vi "New User (popup).vi"(0 "file path (use dialog)":path, 11 "error in (no error)":errorcluster) -> (15 "error out":errorcluster)   [LabVIEW 2012]
uses:
  SubVIs/typedef/User Accounts.ctl
panel:
  out "Info Password not secure":bool
  out "Stop App?":bool
  in  "Cancel":bool
  in  "User\nName":string
  in  "Password":string
  in  "Rewrite\nPassword":string
  in  "Admin":bool
  in  "Create":bool
  # "Log In attempt"
  # "of"
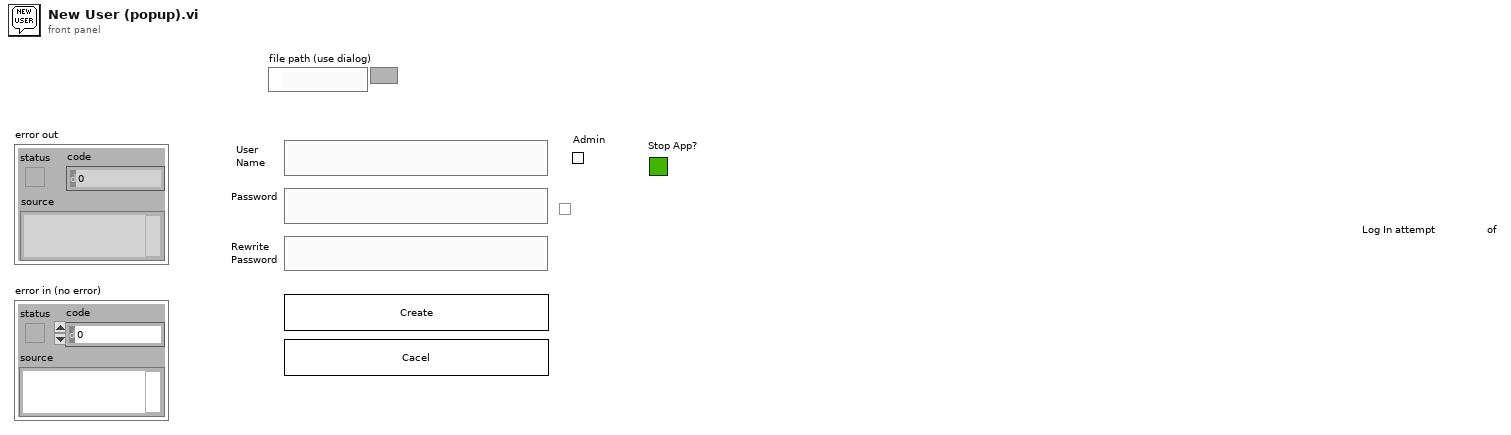
[diagram p1: front panel]
types:
  T1 = typedef "User Accounts.ctl" = enum16{"None", "User", "Admin"}
  T2 = cluster{"Usuario":string, "Password":string, "Account type":T1}
  T3 = typedef "User_Data_Cluster.ctl" = cluster{"Usuario":string, "Password":string, "Account type":T1, "Time Stamp":timestamp}
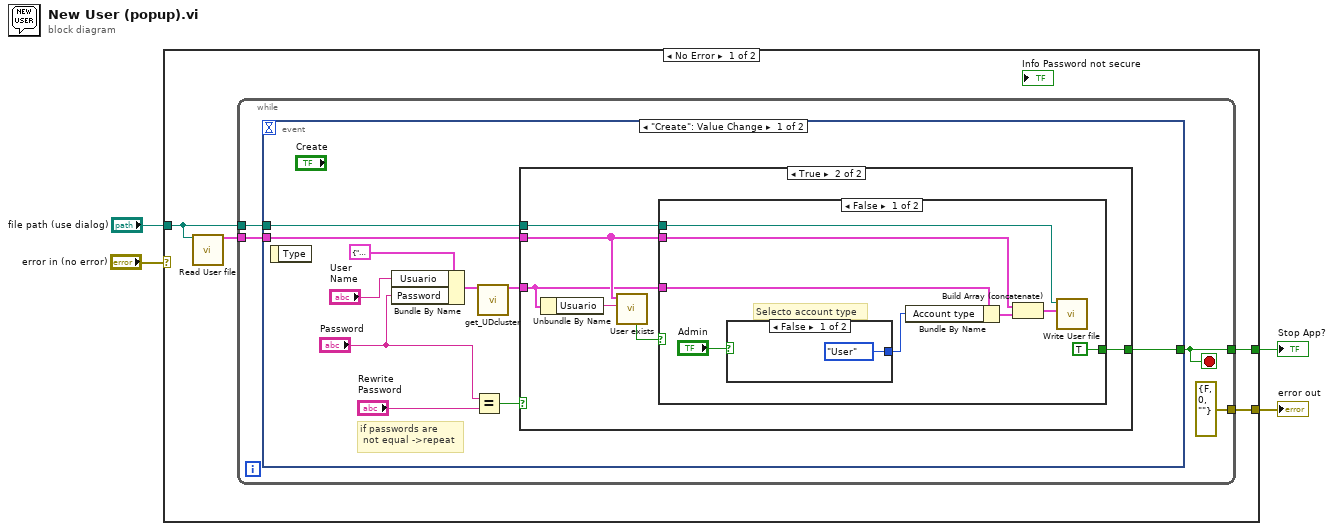
[diagram p0: block diagram]
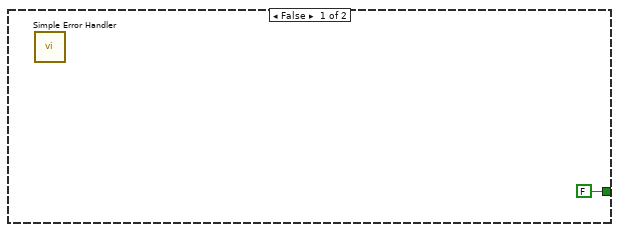
[diagram p2: hidden frame]
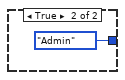
[diagram p3: hidden frame]
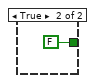
[diagram p4: hidden frame]
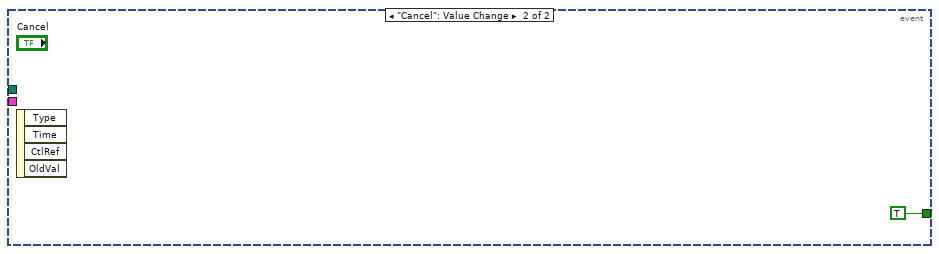
[diagram p5: hidden frame]
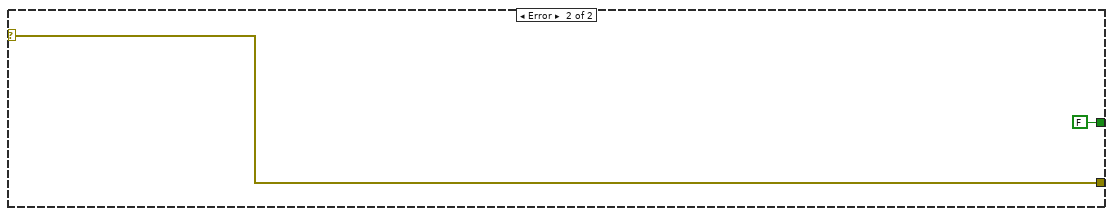
[diagram p6: hidden frame]
diagram:
  n1 = case shown="No Error" "error in (no error)" {
    selector: "error in (no error)" -> [_ w43]
    tunnel: [w8 FALSE] -> w4
    tunnel: [w7 w43] -> w3
    tunnel: "file path (use dialog)" -> [w5 _]
    frame No Error {
      n2 = call "Read User file.vi"("file path (use dialog)"=w5) -> ("Array"=w6:T3[])  [unwired: 13 in, 1 out]
      n3 = while {
        tunnel: [w10] -> w8
        tunnel: [errorcluster {"status"=FALSE, "code"=0, "source"=""} ("error in (no error)")] -> w7
        tunnel: w6 -> [w12]
        tunnel: w5 -> [w11]
        stop <- w10 stop-if-true
        n4 = event shown="[0] \"Create\": Value Change" {
          selector: _ -> [_ _]
          dyn-events: _ -> [_ _]
          timeout: _ -> [_ _]
          tunnel: w12 -> [w21 _]
          tunnel: w11 -> [w22 _]
          tunnel: [w15 TRUE] -> w10
          event "Create": Value Change {
            # "if passwords are\n not equal ->repeat"
            n5 = event-data() -> ()  [unwired: 1 in, 1 out]
            n6 = Bundle By Name(cluster=T2 {"Usuario"="", "Password"="", "Account type"=enum."None"} ("Data imput"), "Usuario"="User\nName", "Password"="Password") -> (w14:T2)
            n7 = Equal?(x="Password", y="Rewrite\nPassword") -> (x = y?=w16:bool)
            n8 = call "get_UDcluster.vi"("Cluster"=w14) -> ("User-data cluster out"=w13:T3)  [unwired: 13 in, 1 out]
            n9 = case shown="True" w16 {
              tunnel: w22 -> [_ w29]
              tunnel: w21 -> [_ w27]
              tunnel: w13 -> [_ w26]
              tunnel: [FALSE w24] -> w15
              frame False {
                n10 = call <vilib>:"Simple Error Handler.vi"() -> ()  [unwired: 5 in, 5 out]
              }
              frame True {
                n11 = Unbundle By Name(w26) -> ("Usuario"=w28:string)
                n12 = call "User exists.vi"("user"=w28, "Array"=w27) -> ("exist?"=w25:bool)  [unwired: 6 in, 3 out]
                n13 = case shown="False" w25 {
                  tunnel: w29 -> [w35 _]
                  tunnel: w26 -> [w30 _]
                  tunnel: w27 -> [w33 _]
                  tunnel: [TRUE FALSE] -> w24
                  frame False {
                    # "Selecto account type"
                    n14 = case shown="False" "Admin" {
                      tunnel: [User_Accounts."User" ("Account") User_Accounts."Admin" ("Account 2")] -> w36
                      frame False {
                      }
                      frame True {
                      }
                    }
                    n15 = Bundle By Name(cluster=w30, "Account type"=w36) -> (w32:T3)
                    n16 = Build Array (concatenate)(w33, w32) -> (w34:T3[])
                    n17 = call "Write User file.vi"("Array"=w34, "file path (use dialog)"=w35) -> ()  [unwired: 8 in, 2 out]
                  }
                  frame True {
                  }
                }
              }
            }
          }
          event "Cancel": Value Change {
            n18 = event-data() -> ()  [unwired: 1 in, 4 out]
          }
        }
      }
    }
    frame Error {
    }
  }
  "error out" <- w3
  "Stop App?" <- w4
